vi "Get Uim Dev Info wrapper.vi"(8 "error in (no error)":errorcluster caption="错误输入（无错误）", 9 "pszDevName":string, 10 "pDummyDevInfoObj":T2, 11 "dwDevIndex":u32) -> (0 "error out":errorcluster caption="错误输出", 1 "DEV_INFO_OBJ":T1, 3 "function return":u32)   [LabVIEW 2016, in "UISimCanFunc_wrapper.lvlib"]
doc: "_declspec (dllexport) DWORD GetUimDevInfo_wrapper(DWORD dwDevIndex, P_DUMMY_DEV_INFO_OBJ pDummyDevInfoObj, CHAR pszDevName[64]);"
uses:
  <userlib>/UISimCanFunc_wrapper/UISimCanFunc_wrapper.lvlib
  <userlib>/UISimCanFunc_wrapper/ctl/DEV_INFO_OBJ.ctl
  <userlib>/UISimCanFunc_wrapper/UISimCanFunc_wrapper.dll
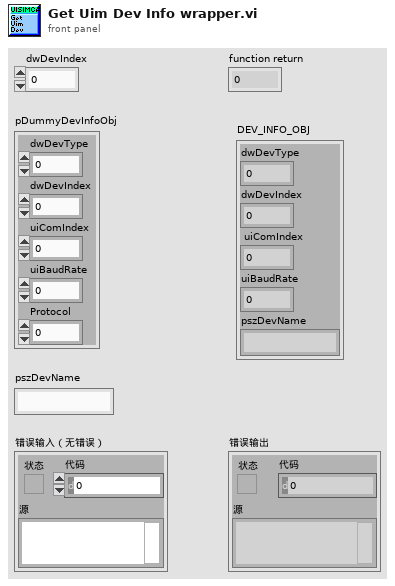
[diagram p1: front panel]
types:
  T1 = typedef "UISimCanFunc_wrapper.lvlib/DEV_INFO_OBJ.ctl" = cluster{"dwDevType":u32, "dwDevIndex":u32, " uiComIndex":u32, "uiBaudRate":u32, "pszDevName":string}
  T2 = cluster{"dwDevType":u32, "dwDevIndex":u32, "uiComIndex":u32, "uiBaudRate":u32, "Protocol":u32}
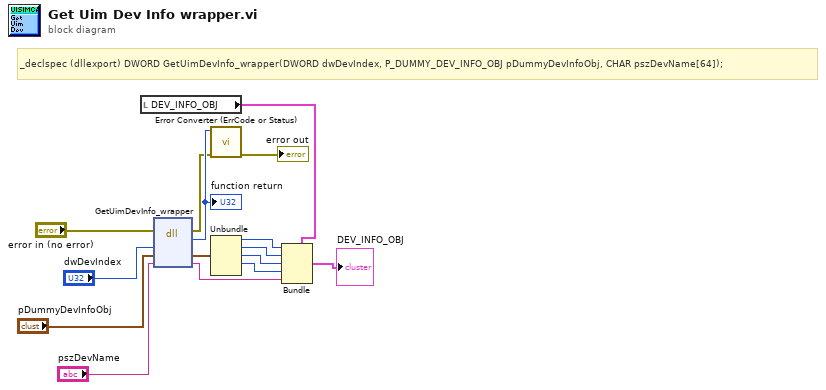
[diagram p0: block diagram]
diagram:
  # "_declspec (dllexport) DWORD GetUimDevInfo_wrapper(DWORD dwDevIndex, P_DUMMY_DEV_INFO_OBJ pDummyDevInfoObj, CHAR pszDevName[64]);"
  n1 = local read "DEV_INFO_OBJ"() -> (w8:T1)
  n2 = dll-call lib="C:/Program Files (x86)/National Instruments/LabVIEW 2016/user.lib/UISimCanFunc_wrapper/UISimCanFunc_wrapper.*" fn="GetUimDevInfo_wrapper"(error in="error in (no error)", "dwDevIndex"="dwDevIndex", "pDummyDevInfoObj"="pDummyDevInfoObj", "pszDevName"="pszDevName") -> (error out=w10:errorcluster, w15:u32, "pDummyDevInfoObj"=w5:T2, "pszDevName"=w6:string)  [unwired: 3 in, 1 out]
  "function return" <- w15
  n3 = call <userlib>:"Error Converter (ErrCode or Status).vi"("error in (no error)"=w10, "error code"=w15) -> ("error out"=→"error out":errorcluster)  [unwired: 9 in]
  n4 = Unbundle(w5) -> ("dwDevType"=w4:u32, "dwDevIndex"=w3:u32, "uiComIndex"=w2:u32, "uiBaudRate"=w1:u32)  [unwired: 1 out]
  n5 = Bundle(cluster=w8, "dwDevType"=w4, "dwDevIndex"=w3, "uiComIndex"=w2, "uiBaudRate"=w1, "pszDevName"=w6) -> (→"DEV_INFO_OBJ":T1)
